vi "Edge-Tri intersection test.vi"(2 "Triangle":T1, 3 "Edge vector (not unit)":sgl[](array[numeric]), 4 "Edge start point":sgl[](array[numeric])) -> (0 "Intersection point":sgl[](array[numeric]), 1 "Intersection":bool)   [LabVIEW 2014]
uses:
  Typedefs/Triangle.ctl
panel:
  # "PN 13/01/2015"
  # "Vertices"
  # "Edges"
  # "Unit normal"
  # "pre-store"
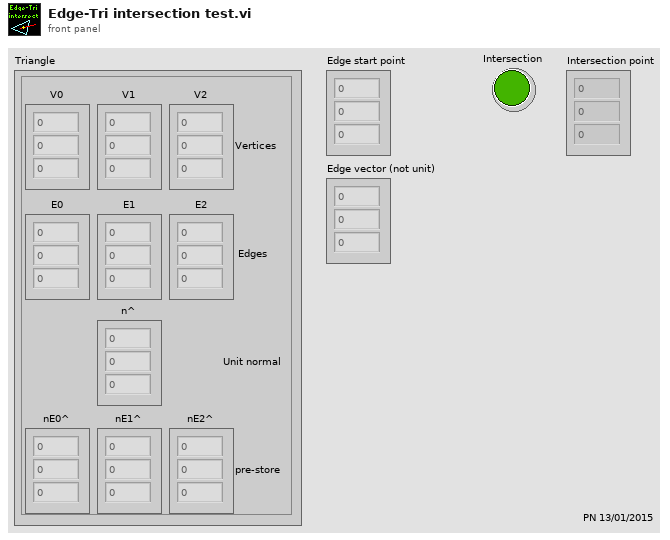
[diagram p1: front panel]
types:
  T1 = typedef "Triangle.ctl" = cluster{"V0":sgl[], "V1":sgl[], "V2":sgl[], "E0":sgl[], "E1":sgl[], "E2":sgl[], "n^":sgl[], "nE0^":sgl[], "nE1^":sgl[], "nE2^":sgl[]}
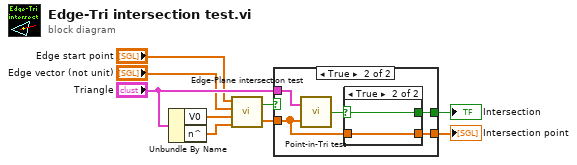
[diagram p0: block diagram]
diagram:
  n1 = Unbundle By Name("Triangle") -> ("V0"=w7:sgl[], "n^"=w8:sgl[])
  n2 = call "Edge-Plane intersection test.vi"("Plane normal (unit)"=w8, "Point on plane"=w7, "Edge vector (not unit)"="Edge vector (not unit)", "Edge start point"="Edge start point") -> ("Intersection point"=w6:sgl[], "Intersection"=w5:bool)
  n3 = case shown="True" w5 {
    selector: w5 -> [w10 _]
    tunnel: w6 -> [_ w13]
    tunnel: "Triangle" -> [_ w15]
    tunnel: [w10 w12] -> w2
    tunnel: [_ w11] -> w1
    frame False {
    }
    frame True {
      n4 = call "Point-in-Tri test.vi"("Point"=w13, "Triangle"=w15) -> ("Point is inside triangle"=w14:bool)
      n5 = case shown="True" w14 {
        selector: w14 -> [w16 w18]
        tunnel: w13 -> [_ w17]
        tunnel: [w16 w18] -> w12
        tunnel: [_ w17] -> w11
        frame False {
        }
        frame True {
        }
      }
    }
  }
  "Intersection" <- w2
  "Intersection point" <- w1
